vi "dealWithSNType.vi"(2 "SNXn":string="49", 3 "SNType":string="LR(YMD1)(D41)", 4 "TimeInput":timestamp=timestamp(3528403701.661259 s since 1904-01-01)) -> (0 "show_str_SNwithWholeFormat":string="LR5AN0021", 1 "legal":bool=TRUE)   [LabVIEW 2011]
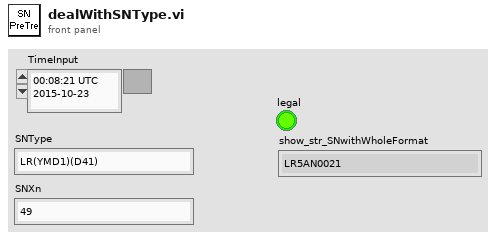
[diagram p1: front panel]
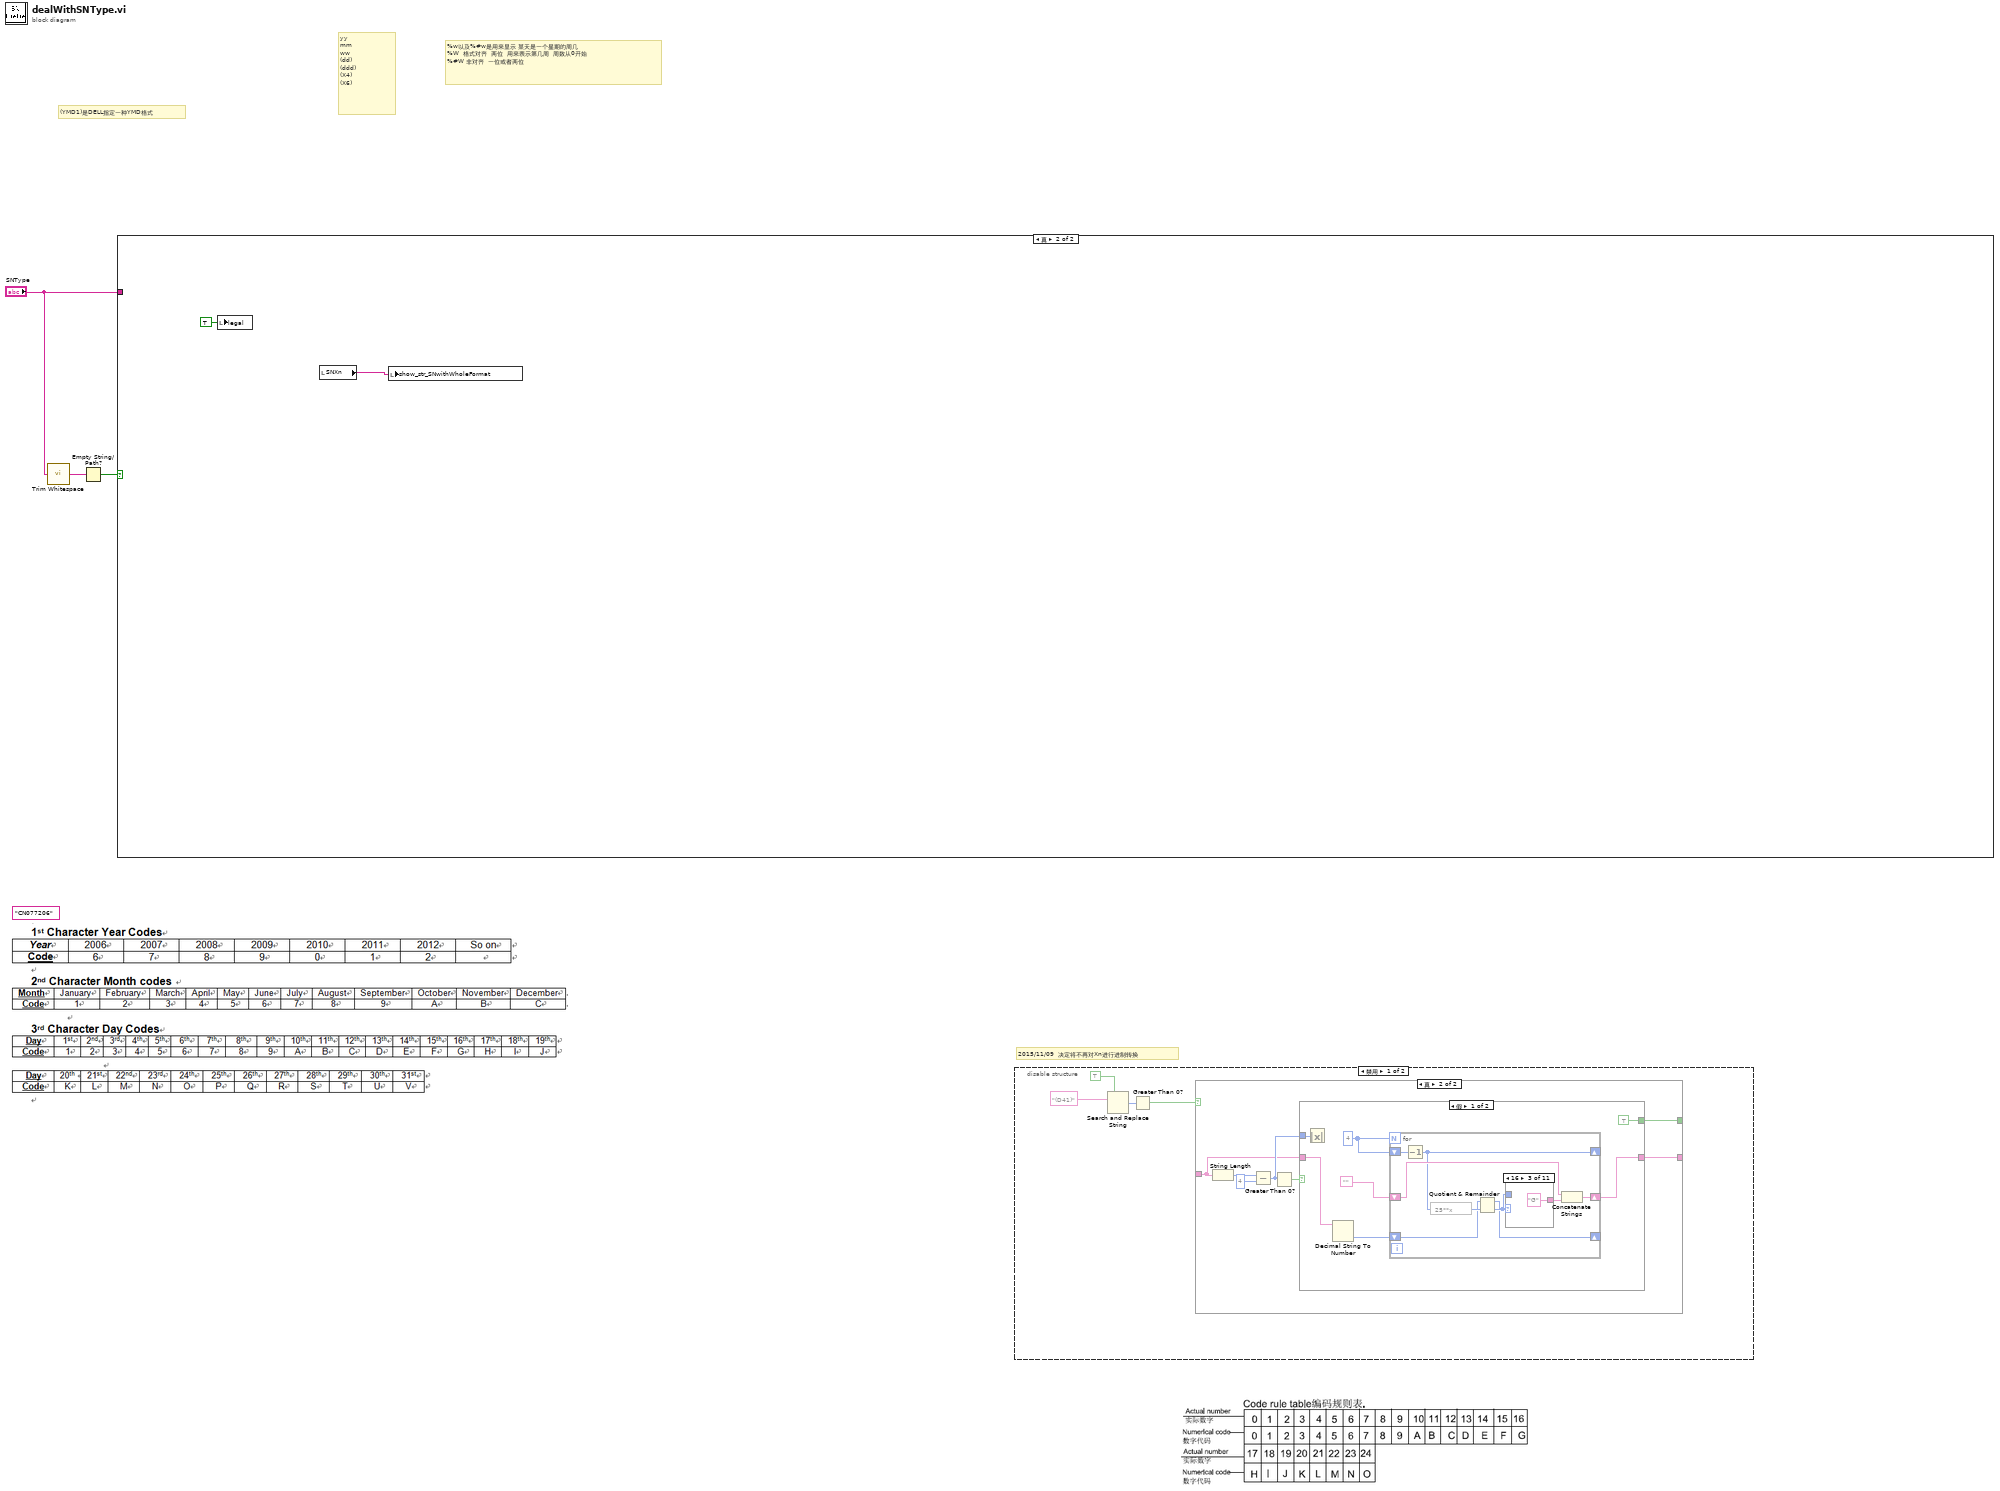
[diagram p0: block diagram]
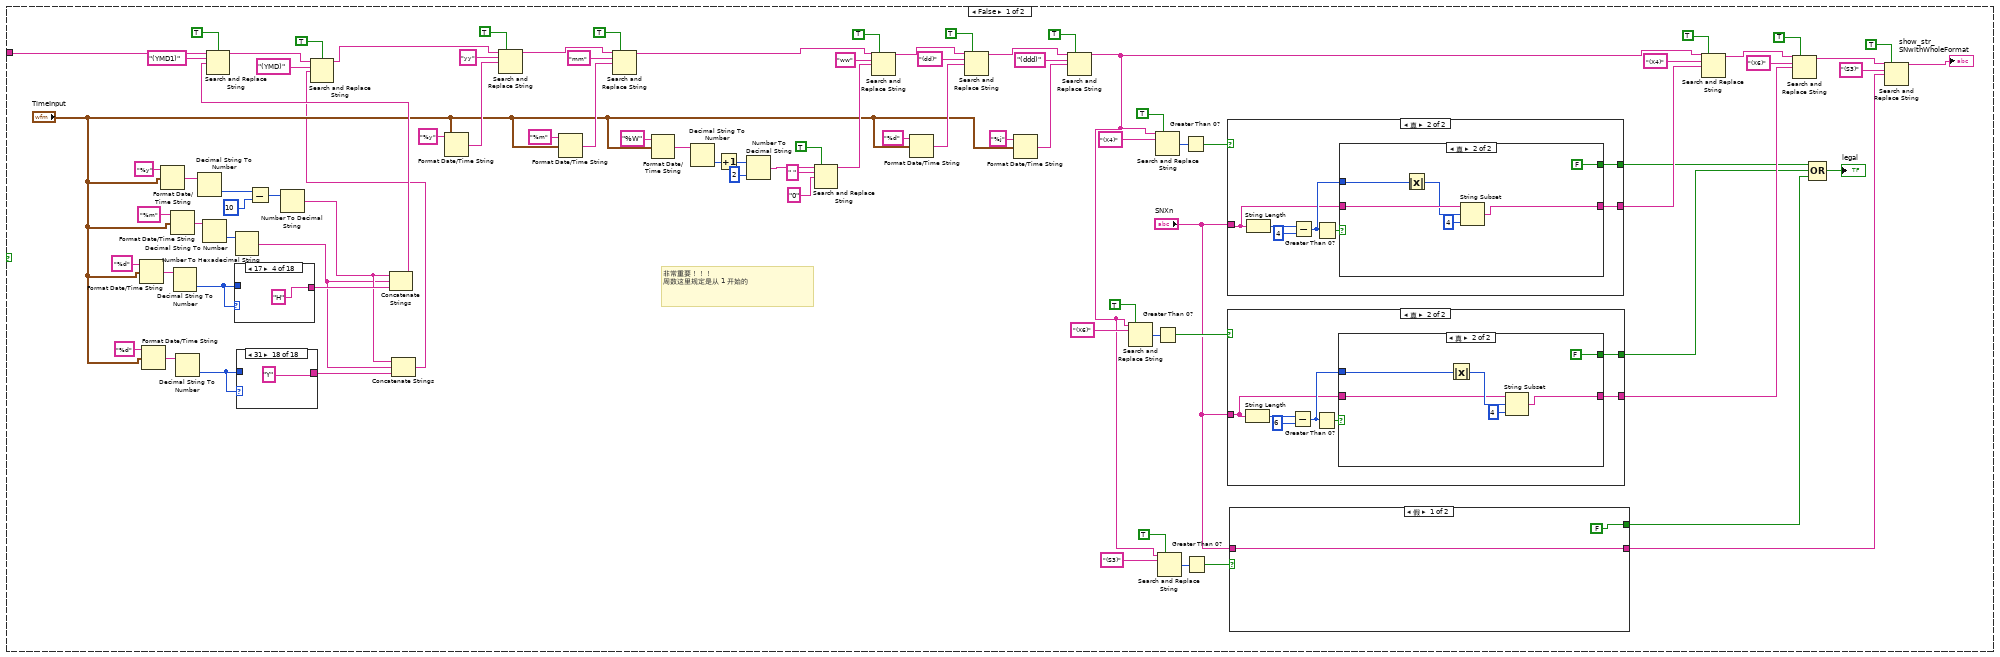
[diagram p2: hidden frame]
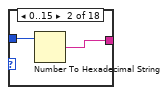
[diagram p4: hidden frame]
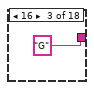
[diagram p5: hidden frame]
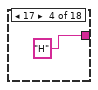
[diagram p6: hidden frame]
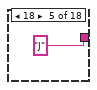
[diagram p7: hidden frame]
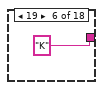
[diagram p8: hidden frame]
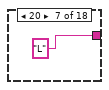
[diagram p9: hidden frame]
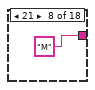
[diagram p10: hidden frame]
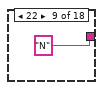
[diagram p11: hidden frame]
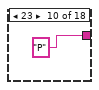
[diagram p12: hidden frame]
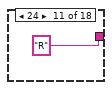
[diagram p13: hidden frame]
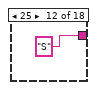
[diagram p14: hidden frame]
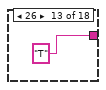
[diagram p15: hidden frame]
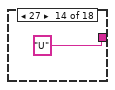
[diagram p16: hidden frame]
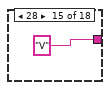
[diagram p17: hidden frame]
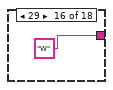
[diagram p18: hidden frame]
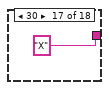
[diagram p19: hidden frame]
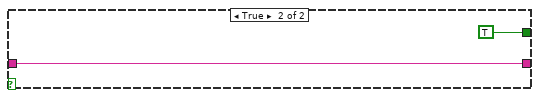
[diagram p20: hidden frame]
diagram:
  (unwired) "CN077206"
  # "2015/11/09  决定将不再对Xn进行进制转换"
  # "(YMD1)是DELL指定一种YMD格式"
  # "%w以及%#w是用来显示 某天是一个星期的周几\n%W  格式对齐  两位  用来表示第几周  周数从0开始\n%#W 非对齐  一位或者两位"
  # "yy\nmm\nww\n(dd)\n(ddd)\n(X4)\n(X6)"
  n1 = call <vilib>:"Trim Whitespace.vi"("string"="SNType") -> ("trimmed string"=w2:string)  [unwired: 1 in]
  n2 = Empty String/Path?(string/path=w2) -> (empty?=w1:bool)
  n3 = case shown="真" w1 {
    tunnel: "SNType" -> [w31 _]
    frame False {
      # "非常重要！！！\n周数这里规定是从 1 开始的"
      n4 = Format Date/Time String(time format string (%c)="%d" ("时间格式字符串(%c)"), seconds (now)="TimeInput") -> (date/time string=w39:string)  [unwired: 1 in]
      n5 = Format Date/Time String(time format string (%c)="%d" ("时间格式字符串(%c)"), seconds (now)="TimeInput") -> (date/time string=w14:string)  [unwired: 1 in]
      n6 = Format Date/Time String(time format string (%c)="%y" ("时间格式字符串(%c)"), seconds (now)="TimeInput") -> (date/time string=w37:string)  [unwired: 1 in]
      n7 = Format Date/Time String(time format string (%c)="%m" ("时间格式字符串(%c)"), seconds (now)="TimeInput") -> (date/time string=w41:string)  [unwired: 1 in]
      n8 = Decimal String To Number(string=w39) -> (number=w33:i32)  [unwired: 2 in, 1 out]
      n9 = Decimal String To Number(string=w14) -> (number=w15:i32)  [unwired: 2 in, 1 out]
      n10 = Decimal String To Number(string=w37) -> (number=w35:i32)  [unwired: 2 in, 1 out]
      n11 = Decimal String To Number(string=w41) -> (number=w40:i32)  [unwired: 2 in, 1 out]
      n12 = case shown="17" w33 {
        tunnel: w33 -> [_ w117 _ _ _ _ _ _ _ _ _ _ _ _ _ _ _ _]
        tunnel: [_ w116 "G" "H" "I" "J" "K" "L" "M" "N" "O" "P" "Q" "R" "S" "T" "U" "V"] -> w32
        frame Default {
        }
        frame 0..15 {
          n13 = Number To Hexadecimal String(2:w117) -> (0:w116:string)  [unwired: 1 in]
        }
        frame 16 {
        }
        frame 17 {
        }
        frame 18 {
        }
        frame 19 {
        }
        frame 20 {
        }
        frame 21 {
        }
        frame 22 {
        }
        frame 23 {
        }
        frame 24 {
        }
        frame 25 {
        }
        frame 26 {
        }
        frame 27 {
        }
        frame 28 {
        }
        frame 29 {
        }
        frame 30 {
        }
        frame 31 {
        }
      }
      n14 = Number To Hexadecimal String(2:w40) -> (0:w10:string)  [unwired: 1 in]
      n15 = case shown="31" w15 {
        tunnel: w15 -> [_ w95 _ _ _ _ _ _ _ _ _ _ _ _ _ _ _ _]
        tunnel: [_ w94 "G" "H" "J" "K" "L" "M" "N" "P" "R" "S" "T" "U" "V" "W" "X" "Y"] -> w16
        frame Default {
        }
        frame 0..15 {
          n16 = Number To Hexadecimal String(2:w95) -> (0:w94:string)  [unwired: 1 in]
        }
        frame 16 {
        }
        frame 17 {
        }
        frame 18 {
        }
        frame 19 {
        }
        frame 20 {
        }
        frame 21 {
        }
        frame 22 {
        }
        frame 23 {
        }
        frame 24 {
        }
        frame 25 {
        }
        frame 26 {
        }
        frame 27 {
        }
        frame 28 {
        }
        frame 29 {
        }
        frame 30 {
        }
        frame 31 {
        }
      }
      n17 = Subtract(x=w35, y=10) -> (x-y=w34:i32)
      n18 = Number To Decimal String(number=w34) -> (decimal integer string=w11:string)  [unwired: 1 in]
      n19 = Concatenate Strings(w11, w10, w32) -> (w29:string)
      n20 = Search and Replace String(case sensitive?=TRUE ("忽略大小写？(F)"), input string=w31, search string="(YMD1)" ("搜索字符串"), replace string=w29) -> (result string=w8:string)  [unwired: 4 in, 3 out]
      n21 = Concatenate Strings(w11, w10, w16) -> (w6:string)
      n22 = Search and Replace String(case sensitive?=TRUE ("忽略大小写？(F)"), input string=w8, search string="(YMD)" ("搜索字符串"), replace string=w6) -> (result string=w7:string)  [unwired: 4 in, 3 out]
      n23 = Format Date/Time String(time format string (%c)="%y" ("时间格式字符串(%c)"), seconds (now)="TimeInput") -> (date/time string=w91:string)  [unwired: 1 in]
      n24 = Search and Replace String(replace all?=TRUE ("替换全部？(F)"), input string=w7, search string="yy" ("搜索字符串"), replace string=w91) -> (result string=w85:string)  [unwired: 4 in, 3 out]
      n25 = Format Date/Time String(time format string (%c)="%m" ("时间格式字符串(%c)"), seconds (now)="TimeInput") -> (date/time string=w88:string)  [unwired: 1 in]
      n26 = Search and Replace String(replace all?=TRUE ("替换全部？(F)"), input string=w85, search string="mm" ("搜索字符串"), replace string=w88) -> (result string=w54:string)  [unwired: 4 in, 3 out]
      n27 = Format Date/Time String(time format string (%c)="%W" ("时间格式字符串(%c)"), seconds (now)="TimeInput") -> (date/time string=w52:string)  [unwired: 1 in]
      n28 = Decimal String To Number(string=w52) -> (number=w51:i32)  [unwired: 2 in, 1 out]
      n29 = Increment(x=w51) -> (x+1=w50:i32)
      n30 = Number To Decimal String(number=w50, width (-)=i16 2 ("宽度(-)")) -> (decimal integer string=w48:string)
      n31 = Search and Replace String(replace all?=TRUE ("替换全部？(F)"), input string=w48, search string=" " ("搜索字符串"), replace string="0" ("替换字符串(\"\")")) -> (result string=w45:string)  [unwired: 4 in, 3 out]
      n32 = Search and Replace String(replace all?=TRUE ("替换全部？(F)"), input string=w54, search string="ww" ("搜索字符串"), replace string=w45) -> (result string=w53:string)  [unwired: 4 in, 3 out]
      n33 = Format Date/Time String(time format string (%c)="%d" ("时间格式字符串(%c)"), seconds (now)="TimeInput") -> (date/time string=w82:string)  [unwired: 1 in]
      n34 = Search and Replace String(replace all?=TRUE ("替换全部？(F)"), input string=w53, search string="(dd)" ("搜索字符串"), replace string=w82) -> (result string=w76:string)  [unwired: 4 in, 3 out]
      n35 = Format Date/Time String(time format string (%c)="%j" ("时间格式字符串(%c)"), seconds (now)="TimeInput") -> (date/time string=w79:string)  [unwired: 1 in]
      n36 = Search and Replace String(replace all?=TRUE ("替换全部？(F)"), input string=w76, search string="(ddd)" ("搜索字符串"), replace string=w79) -> (result string=w25:string)  [unwired: 4 in, 3 out]
      n37 = Search and Replace String(replace all?=TRUE ("替换全部？(F)"), input string=w25, search string="(X6)" ("搜索字符串")) -> (number of replacements=w66:i32)  [unwired: 5 in, 3 out]
      n38 = Search and Replace String(replace all?=TRUE ("替换全部？(F)"), input string=w25, search string="(X4)" ("搜索字符串")) -> (number of replacements=w68:i32)  [unwired: 5 in, 3 out]
      n39 = Greater Than 0?(x=w66) -> (x > 0?=w63:bool)
      n40 = Search and Replace String(replace all?=TRUE ("替换全部？(F)"), input string=w25, search string="(S3)" ("搜索字符串")) -> (number of replacements=w26:i32)  [unwired: 5 in, 3 out]
      n41 = Greater Than 0?(x=w68) -> (x > 0?=w67:bool)
      n42 = Greater Than 0?(x=w26) -> (x > 0?=w24:bool)
      n43 = case shown="真" w63 {
        tunnel: "SNXn" -> [w134 w138]
        tunnel: [w134 w137] -> w61
        tunnel: [FALSE w136] -> w59
        frame False {
        }
        frame True {
          n44 = String Length(string=w138) -> (length=w139:i32)
          n45 = Subtract(x=w139, y=6) -> (x-y=w142:i32)
          n46 = Greater Than 0?(x=w142) -> (x > 0?=w141:bool)
          n47 = case shown="真" w141 {
            tunnel: w142 -> [w147 w152]
            tunnel: w138 -> [w146 w151]
            tunnel: [TRUE FALSE] -> w136
            tunnel: [w144 w153] -> w137
            frame False {
              n48 = Absolute Value(x=w147) -> (abs(x)=w143:i32)
              n49 = for {
                N: w143 -> [_]
                shift-right: [w148] -> w144
                shift-left: w146 -> [w149]
                n50 = Concatenate Strings("0", w149) -> (w148:string)
              }
            }
            frame True {
              n51 = Absolute Value(x=w152) -> (abs(x)=w155:i32)
              n52 = String Subset(string=w151, offset (0)=w155, length (rest)=4 ("长度（剩余）")) -> (substring=w153:string)
            }
          }
        }
      }
      n53 = case shown="真" w67 {
        tunnel: "SNXn" -> [w157 w161]
        tunnel: [w157 w160] -> w62
        tunnel: [FALSE w159] -> w60
        frame False {
        }
        frame True {
          n54 = String Length(string=w161) -> (length=w162:i32)
          n55 = Subtract(x=w162, y=4) -> (x-y=w165:i32)
          n56 = Greater Than 0?(x=w165) -> (x > 0?=w164:bool)
          n57 = case shown="真" w164 {
            tunnel: w165 -> [w170 w176]
            tunnel: w161 -> [w169 w178]
            tunnel: [TRUE FALSE] -> w159
            tunnel: [w167 w177] -> w160
            frame False {
              n58 = Absolute Value(x=w170) -> (abs(x)=w166:i32)
              n59 = for {
                N: w166 -> [_]
                shift-right: [w171] -> w167
                shift-left: w169 -> [w172]
                n60 = Concatenate Strings("0", w172) -> (w171:string)
              }
            }
            frame True {
              n61 = Absolute Value(x=w176) -> (abs(x)=w175:i32)
              n62 = String Subset(string=w178, offset (0)=w175, length (rest)=4 ("长度（剩余）")) -> (substring=w177:string)
            }
          }
        }
      }
      n63 = case shown="假" w24 {
        tunnel: "SNXn" -> [w113 w115]
        tunnel: [w113 w115] -> w17
        tunnel: [FALSE TRUE] -> w22
        frame False {
        }
        frame True {
        }
      }
      n64 = Search and Replace String(replace all?=TRUE ("替换全部？(F)"), input string=w25, search string="(X4)" ("搜索字符串"), replace string=w62) -> (result string=w71:string)  [unwired: 4 in, 3 out]
      n65 = Search and Replace String(replace all?=TRUE ("替换全部？(F)"), input string=w71, search string="(X6)" ("搜索字符串"), replace string=w61) -> (result string=w19:string)  [unwired: 4 in, 3 out]
      n66 = Compound Arithmetic op=OR(w60, w59, w22) -> (→"legal":bool)
      n67 = Search and Replace String(replace all?=TRUE ("替换全部？(F)"), input string=w19, search string="(S3)" ("搜索字符串"), replace string=w17) -> (result string=→"show_str_SNwithWholeFormat":string)  [unwired: 4 in, 3 out]
    }
    frame True {
      n68 = local write "legal"(TRUE ("legal")) -> ()
      n69 = local read "SNXn"() -> (w180:string)
      n70 = local write "show_str_SNwithWholeFormat"(w180) -> ()
    }
  }
  n71 = disable-structure shown="禁用" {
    frame Disabled {
      n72 = Search and Replace String(replace all?=TRUE ("替换全部？(F)"), search string="(D41)" ("搜索字符串")) -> (number of replacements=w182:i32)  [unwired: 6 in, 3 out]
      n73 = Greater Than 0?(x=w182) -> (x > 0?=w185:bool)
      n74 = case shown="真" w185 {
        tunnel: _ -> [w186 w190]
        tunnel: [w186 w189] -> _
        tunnel: [FALSE w188] -> _
        frame False {
        }
        frame True {
          n75 = String Length(string=w190) -> (length=w191:i32)
          n76 = Subtract(x=w191, y=4) -> (x-y=w194:i32)
          n77 = Greater Than 0?(x=w194) -> (x > 0?=w193:bool)
          n78 = case shown="假" w193 {
            tunnel: w194 -> [w201 _]
            tunnel: w190 -> [w196 w223]
            tunnel: [TRUE FALSE] -> w188
            tunnel: [w195 w223] -> w189
            frame False {
              w198 = 4
              n79 = Absolute Value(x=w201) -> ()  [unwired: 1 out]
              n80 = Decimal String To Number(string=w196) -> (number=w199:i32)  [unwired: 2 in, 1 out]
              n81 = for {
                N: w198 -> [_]
                shift-right: [w206] -> w195
                shift-left: "" -> [w207]
                shift-right: [w204] -> _
                shift-left: w198 -> [w205]
                shift-right: [w202] -> _
                shift-left: w199 -> [w203]
                n82 = Decrement(x=w205) -> (x-1=w204:i32)
                n83 = expression code="25**x"(w204) -> (w210:i32)
                n84 = Quotient & Remainder(x=w203, y=w210) -> (x-y*floor(x/y)=w202:i32, floor(x/y)=w209:i32)
                n85 = case shown="16" w209 {
                  tunnel: w209 -> [_ w212 _ _ _ _ _ _ _ _ _]
                  tunnel: [_ w211 "G" "H" "I" "J" "K" "L" "M" "N" "O"] -> w208
                  frame Default {
                  }
                  frame 0..15 {
                    n86 = Number To Hexadecimal String(2:w212) -> (0:w211:string)  [unwired: 1 in]
                  }
                  frame 16 {
                  }
                  frame 17 {
                  }
                  frame 18 {
                  }
                  frame 19 {
                  }
                  frame 20 {
                  }
                  frame 21 {
                  }
                  frame 22 {
                  }
                  frame 23 {
                  }
                  frame 24 {
                  }
                }
                n87 = Concatenate Strings(w207, w208) -> (w206:string)
              }
            }
            frame True {
              n88 = One Button Dialog(message="流水码位数和标签上选择的位数不一致！\n可能会遗失部分信息，拒绝打印！" ("消息")) -> ()  [unwired: 1 in, 1 out]
            }
          }
        }
      }
    }
    frame Enabled {
    }
  }
